vi "Talker.vi"(0 "Add in":refnum<class "Add.lvclass">, 5 "Subpanel Ref":refnum<vi>, 11 "Error In":errorcluster) -> (4 "Add out":refnum<class "Add.lvclass">, 15 "Error Out":errorcluster)   [LabVIEW 2020, in "Add.lvclass"]
doc: "Method to call the UI Method. This will pass the object to the UI Method which will do the operation and return the object to the main vi."
uses:
  Add.lvclass
  Add.lvclass/Add.ctl
  UI.vi
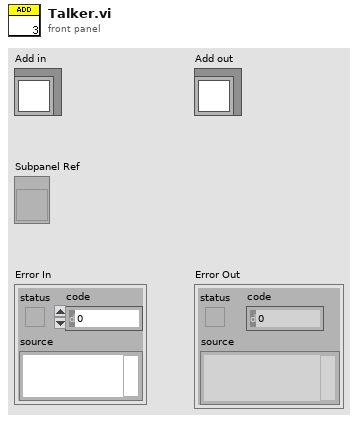
[diagram p1: front panel]
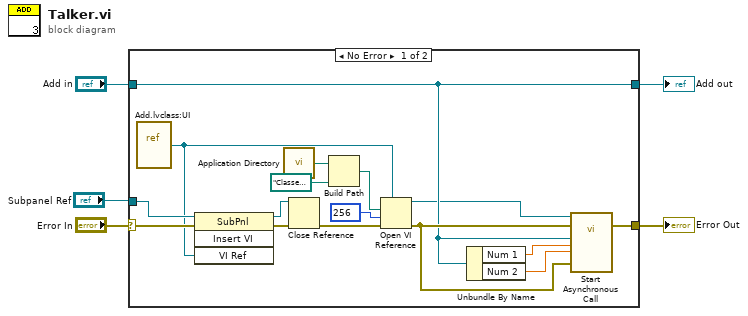
[diagram p0: block diagram]
diagram:
  n1 = case shown="No Error" "Error In" {
    selector: "Error In" -> [w13 w23]
    tunnel: [w18 w23] -> w4
    tunnel: [w17 w22] -> w2
    tunnel: "Add in" -> [w17 w22]
    tunnel: "Subpanel Ref" -> [w11 _]
    frame No Error {
      n2 = vi-ref "Add.lvclass:UI.vi"() -> (w6:refnum<vi>)
      n3 = invoke on="Invoke Node" class="SubPnl" method="Insert VI"(reference=w11, error in=w13, "VI Ref"=w6) -> (reference out=w7:refnum<vi>, error out=w12:errorcluster)  [unwired: 1 in, 2 out]
      n4 = call <vilib>:"Application Directory.vi"() -> ("Application Directory"=w15:path)
      n5 = Close Reference(reference=w7, error in (no error)=w12) -> (error out=w8:errorcluster)
      n6 = Build Path(base path=w15, name or relative path=path "Classes/Children/Add/Methods/UI.vi") -> (appended path=w9:path)
      n7 = Open VI Reference(type specifier VI Refnum (for type only)=w6, vi path=w9, options=256, error in (no error)=w8) -> (vi reference=w10:refnum<vi>, error out=w19:errorcluster)  [unwired: 2 in]
      n8 = Unbundle By Name(w17) -> ("Num 1"=w21:dbl, "Num 2"=w20:dbl)
      n9 = call-by-ref "Start Asynchronous Call"(reference=w10, error in=w19, "Add.lvclass"=w17, "Num 1"=w21, "Num 2"=w20, "Error In"=w19) -> (error out=w18:errorcluster)  [unwired: 9 in, 4 out]
    }
    frame Error {
    }
  }
  "Error Out" <- w4
  "Add out" <- w2
